vi "OutputArm.vi"() -> ()   [LabVIEW 2020]
uses:
  GlobalArm.vi
  TAI_Motor.vi
  GlobalDriverStationData.vi
panel:
  in  "Wrist Torque Compensation":dbl=1.0
  in  "Elbow Torque Compensation":dbl=1.0
  in  "Shoulder Torque Compensation":dbl=1.0
  in  "Shoulder Overrided State":enum16{"Safety", "Travelling", "Positioning"}(ring)
  in  "Elbow Overrided State":enum16{"Safety", "Travelling", "Positioning"}(ring)
  in  "Wrist Overrided State":enum16{"Safety", "Travelling", "Positioning"}(ring)
  in  "Wrist S-Curve Strength":dbl=4.0
  in  "Wrist Acceleration (deg/s^2)":dbl=300.0
  in  "Wrist Cruise Velocity (deg/s)":dbl=60.0
  in  "Wrist Override (deg)":dbl
  in  "Override Wrist State Machine":bool
  out "Wrist Position (deg)":dbl
  out "Wrist Position":cluster{dbl, "Interlock Output":dbl}(graph)
  out "Wrist Velocity":cluster{dbl}(graph)
  in  "Wrist Positioning PID Parameters":T1={"Kp"=0.0, "Ki"=0.0, "Kd"=0.0, "Kf (don't use)"=0.0, "I-Zone"=10.0} {"Kd" min=0.0; "Ki" min=0.0; "Kp" min=0.0}
  in  "Wrist Travelling PID Parameters":T1={"Kp"=0.0, "Ki"=0.0, "Kd"=0.0, "Kf (don't use)"=0.0, "I-Zone"=10.0} {"Kd" min=0.0; "Ki" min=0.0; "Kp" min=0.0}
  in  "Shoulder S-Curve Strength":dbl=4.0
  in  "Shoulder Acceleration (deg/s^2)":dbl=300.0
  in  "Shoulder Cruise Velocity (deg/s)":dbl=60.0
  in  "Shoulder Override (deg)":dbl
  in  "Override Shoulder State Machine":bool
  out "Shoulder Position (deg)":dbl
  out "Shoulder Position":cluster{dbl, "Interlock Output":dbl}(graph)
  out "Shoulder Velocity":cluster{dbl}(graph)
  in  "Shoulder Positioning PID Parameters":T1={"Kp"=0.0, "Ki"=0.0, "Kd"=0.0, "Kf (don't use)"=0.0, "I-Zone"=10.0} {"Kd" min=0.0; "Ki" min=0.0; "Kp" min=0.0}
  in  "Shoulder Travelling PID Parameters":T1={"Kp"=0.0, "Ki"=0.0, "Kd"=0.0, "Kf (don't use)"=0.0, "I-Zone"=10.0} {"Kd" min=0.0; "Ki" min=0.0; "Kp" min=0.0}
  in  "Elbow Override (deg)":dbl
  in  "Override Elbow State Machine":bool
  out "Elbow Position":cluster{dbl, "Interlock Output":dbl}(graph)
  out "Elbow Position (deg)":dbl
  out "Elbow Velocity":cluster{dbl}(graph)
  in  "Plot Joint Positions":bool
  in  "Elbow Positioning PID Parameters":T1={"Kp"=inf, "Ki"=0.0, "Kd"=0.0, "Kf (don't use)"=0.0, "I-Zone"=10.0} {"Kd" min=0.0; "Ki" min=0.0; "Kp" min=0.0}
  in  "Elbow Travelling PID Parameters":T1={"Kp"=0.0, "Ki"=0.0, "Kd"=0.0, "Kf (don't use)"=0.0, "I-Zone"=10.0} {"Kd" min=0.0; "Ki" min=0.0; "Kp" min=0.0}
  in  "Elbow S-Curve Strength":dbl=4.0
  in  "Elbow Acceleration (deg/s^2)":dbl=300.0
  in  "Elbow Cruise Velocity (deg/s)":dbl=60.0
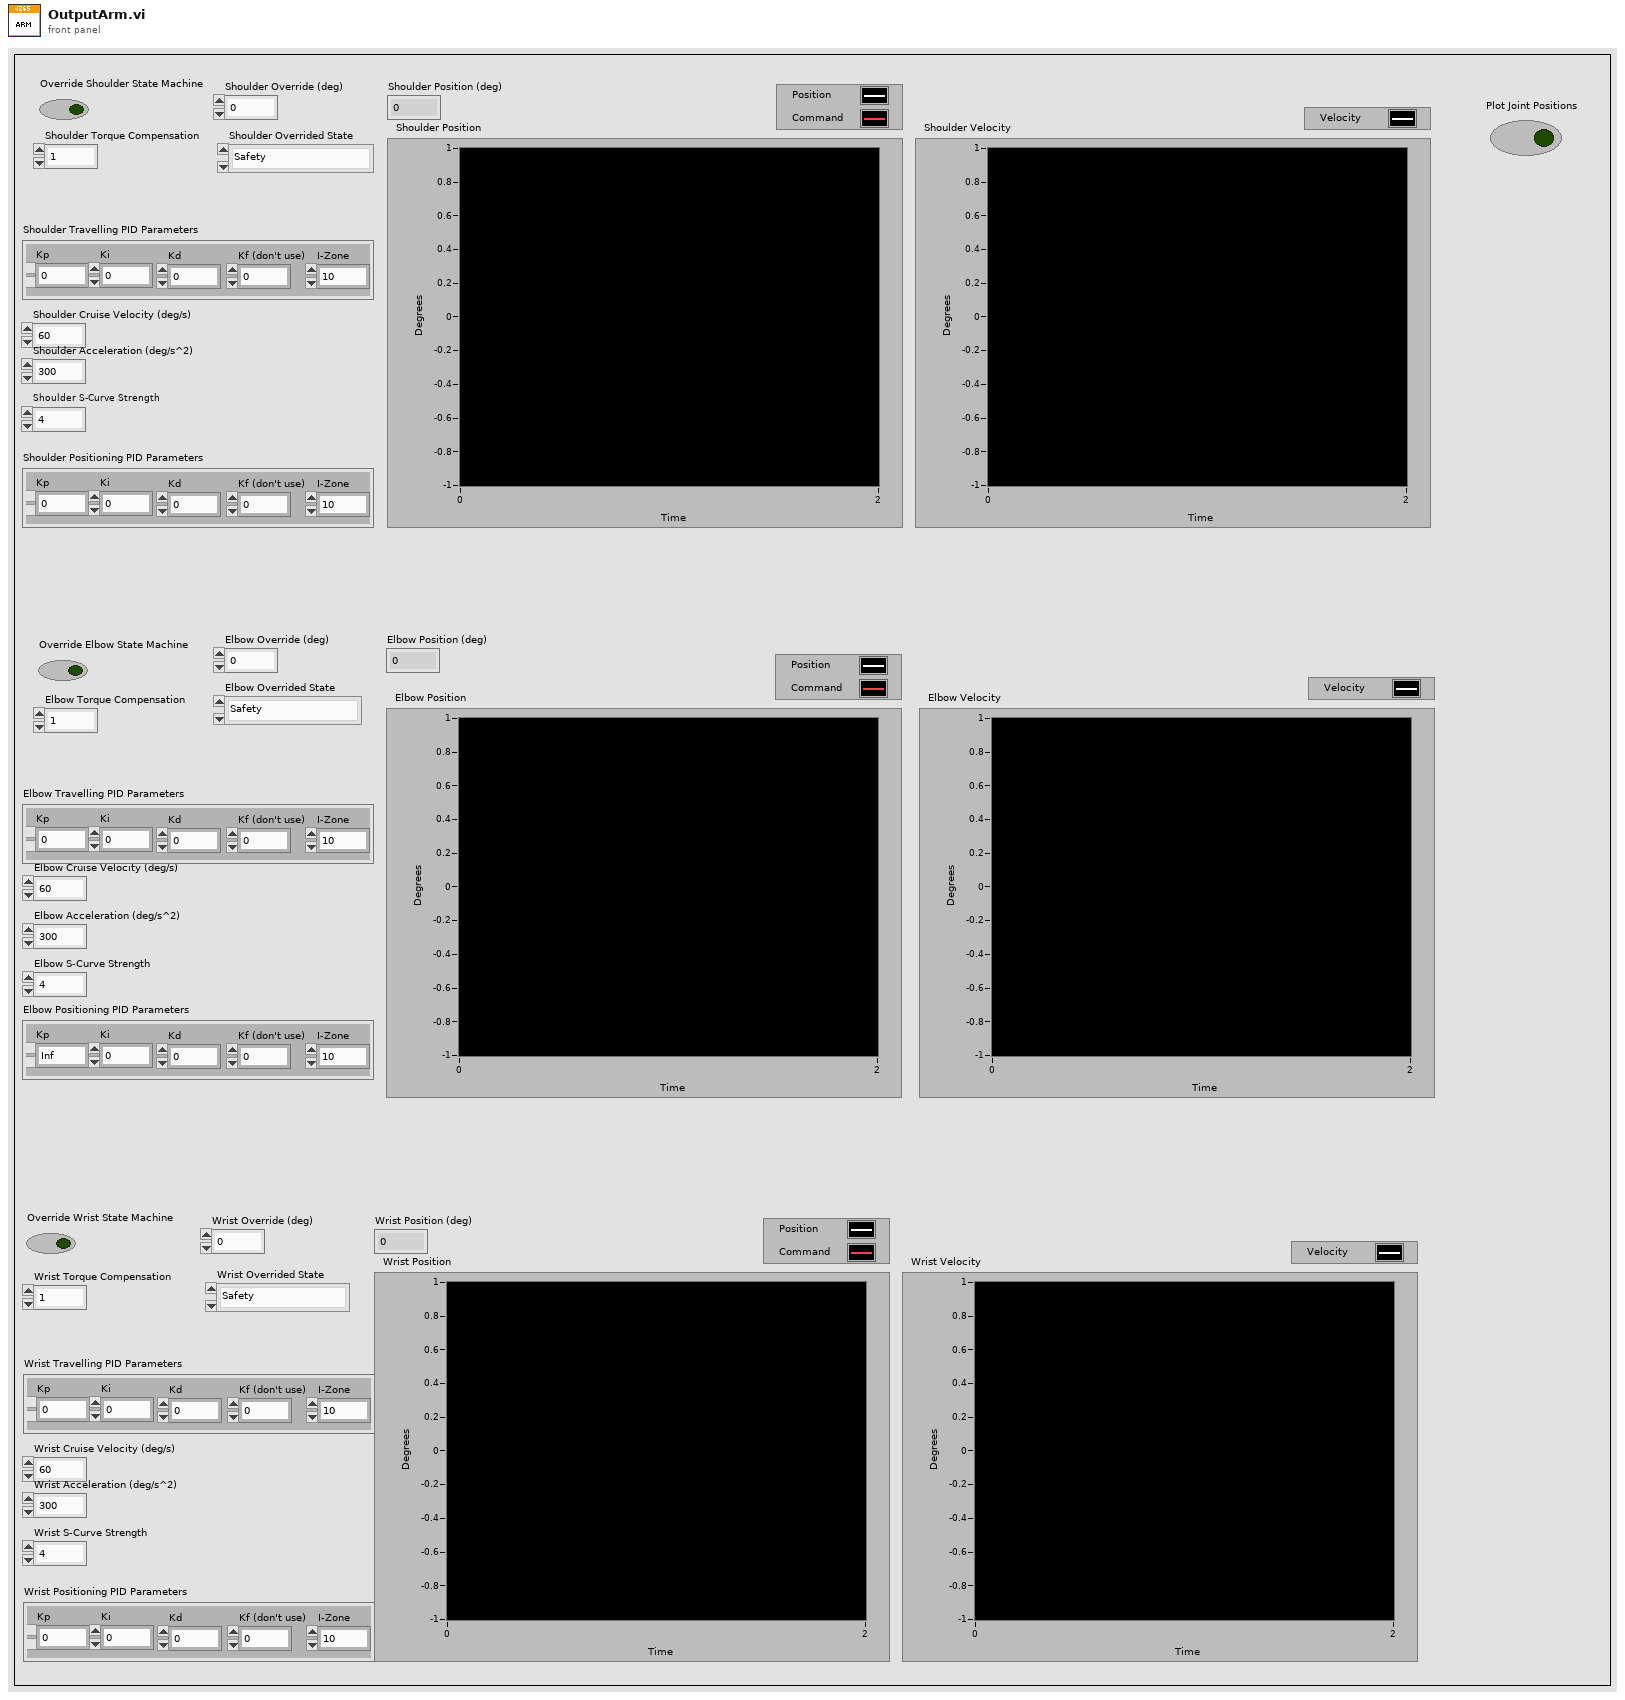
[diagram p1: front panel]
types:
  T1 = cluster{"Kp":dbl, "Ki":dbl, "Kd":dbl, "Kf (don't use)":dbl, "I-Zone":dbl}
  T2 = typedef "WPI_MotorControlDeviceRef.ctl" = cluster{"DeviceStatus":errorcluster, "Type":T3, "PWM":cluster{"PWM Channel":T4, "DeadBand":T5}, "CAN":cluster{"Device Number":u8, "SetOutput VI Ref":variant, "GetOutput VI Ref":variant, "Enable VI Ref":variant, "Disable VI Ref":variant, "Data":variant}, "Invert":bool, "DIO PWM":cluster{"PWM \"Enable\" Channel":T4, "DIOChannel":T6, "PWM Rate":dbl}}
  T3 = typedef "WPI_MotorControlType.ctl" = enum16{"PWM", "CAN", "DIO PWM"}
  T4 = typedef "FPGA_DIOPWMChannel.ctl" = enum8{"PWM 0", "PWM 1", "PWM 2", "PWM 3", "PWM 4", "PWM 5", "PWM 6", "PWM 7", "PWM 8", "PWM 9", "PWM MXP 0", "PWM MXP 1", "PWM MXP 2", "PWM MXP 3", "PWM MXP 4", "PWM MXP 5", "PWM MXP 6", "PWM MXP 7", "PWM MXP 8", "PWM MXP 9", "Invalid"}
  T5 = typedef "WPI_PWMDeadband.ctl" = cluster{"Name":string, "maxPositivePwm":i32, "minPositivePwm":i32, "centerPwm":i32, "maxNegativePwm":i32, "minNegativePwm":i32, "angularRange":u16}
  T6 = typedef "FPGA_DIOChannel.ctl" = enum8{"DIO 0", "DIO 1", "DIO 2", "DIO 3", "DIO 4", "DIO 5", "DIO 6", "DIO 7", "DIO 8", "DIO 9", "DIO MXP 0", "DIO MXP 1", "DIO MXP 2", "DIO MXP 3", "DIO MXP 4", "DIO MXP 5", "DIO MXP 6", "DIO MXP 7", "DIO MXP 8", "DIO MXP 9", "DIO MXP 10", "DIO MXP 11", "DIO MXP 12", "DIO MXP 13", "DIO MXP 14", "DIO MXP 15", "SPI Port CS1", "SPI Port CS2", "SPI Port CS3", "SPI Port MISO", "SPI Port MOSI", "Invalid"}
  T7 = enum16{"No Changed Output", "New Normal Output", "New Testing Output"}
  T8 = cluster{"Position (deg)":dbl, "OUT_Shoulder_Goal (deg)":dbl}
  T9 = cluster{"Position (deg)":dbl, "OUT_Wrist_Goal (deg)":dbl}
  T10 = cluster{"Position (deg)":dbl, "OUT_Elbow_Goal (deg)":dbl}
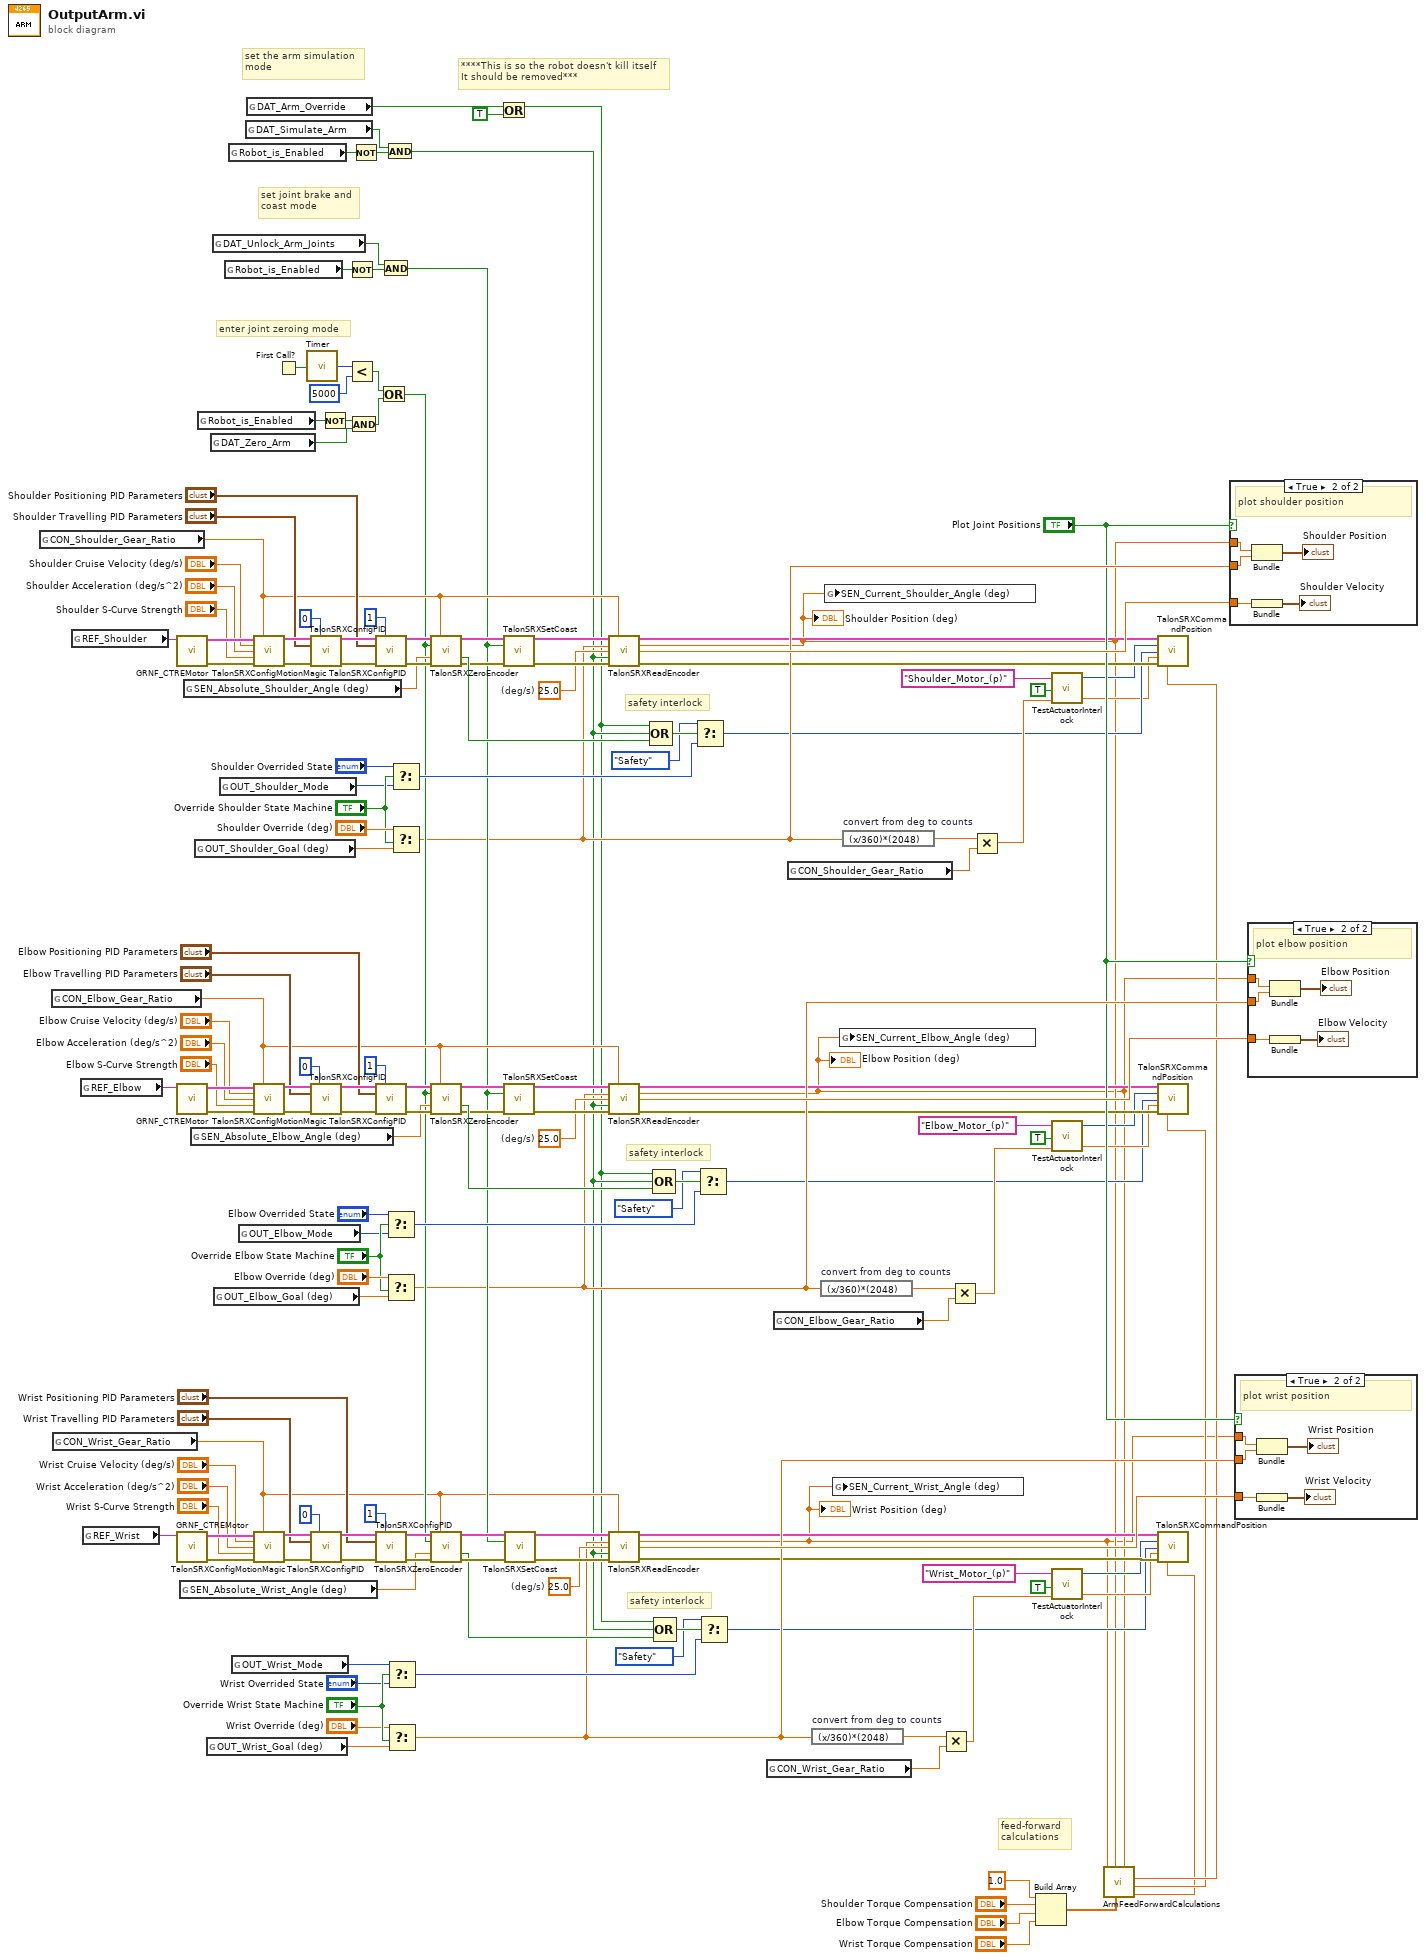
[diagram p0: block diagram]
diagram:
  w39 = 25.0  # (deg/s)
  w91 = 25.0  # (deg/s)
  w113 = 25.0  # (deg/s)
  # "****This is so the robot doesn't kill itself\nIt should be removed***"
  # "feed-forward\ncalculations"
  # "set the arm simulation\nmode"
  # "safety interlock"
  # "safety interlock"
  # "safety interlock"
  # "enter joint zeroing mode"
  # "set joint brake and\ncoast mode"
  n1 = global read "GlobalArm.vi" "CON_Shoulder_Gear_Ratio"() -> (w115:dbl)
  n2 = global read "GlobalArm.vi" "CON_Elbow_Gear_Ratio"() -> (w82:dbl)
  n3 = global read "GlobalArm.vi" "CON_Wrist_Gear_Ratio"() -> (w50:dbl)
  n4 = global read "GlobalArm.vi" "REF_Shoulder"() -> (w162:string)
  n5 = global read "GlobalArm.vi" "REF_Elbow"() -> (w88:string)
  n6 = global read "GlobalArm.vi" "REF_Wrist"() -> (w69:string)
  n7 = call "GRNF_CTREMotor.vi"("RefNum Name"=w162) -> ("Error"=w161:errorcluster, "Device Reference"=w134:T2)  [unwired: 5 in]
  n8 = call "GRNF_CTREMotor.vi"("RefNum Name"=w88) -> ("Error"=w111:errorcluster, "Device Reference"=w104:T2)  [unwired: 5 in]
  n9 = call "GRNF_CTREMotor.vi"("RefNum Name"=w69) -> ("Error"=w67:errorcluster, "Device Reference"=w77:T2)  [unwired: 5 in]
  n10 = global read "GlobalArm.vi" "SEN_Absolute_Wrist_Angle (deg)"() -> (w51:dbl)
  n11 = global read "GlobalArm.vi" "SEN_Absolute_Shoulder_Angle (deg)"() -> (w120:dbl)
  n12 = global read "GlobalArm.vi" "SEN_Absolute_Elbow_Angle (deg)"() -> (w97:dbl)
  n13 = global read "GlobalArm.vi" "OUT_Shoulder_Goal (deg)"() -> (w160:dbl)
  n14 = global read "GlobalDriverStationData.vi" "Robot_is_Enabled"() -> (w151:bool)
  n15 = global read "GlobalArm.vi" "OUT_Wrist_Goal (deg)"() -> (w49:dbl)
  n16 = global read "GlobalArm.vi" "DAT_Zero_Arm"() -> (w143:bool)
  n17 = global read "GlobalArm.vi" "DAT_Unlock_Arm_Joints"() -> (w140:bool)
  n18 = global read "GlobalArm.vi" "OUT_Elbow_Goal (deg)"() -> (w110:dbl)
  n19 = global read "GlobalArm.vi" "OUT_Shoulder_Mode"() -> (w46:enum16{"Safety", "Travelling", "Positioning"})
  n20 = global read "GlobalDriverStationData.vi" "Robot_is_Enabled"() -> (w142:bool)
  n21 = global read "GlobalDriverStationData.vi" "Robot_is_Enabled"() -> (w30:bool)
  n22 = global read "GlobalArm.vi" "OUT_Wrist_Mode"() -> (w41:enum16{"Safety", "Travelling", "Positioning"})
  n23 = global read "GlobalArm.vi" "OUT_Elbow_Mode"() -> (w44:enum16{"Safety", "Travelling", "Positioning"})
  n24 = global read "GlobalArm.vi" "DAT_Simulate_Arm"() -> (w28:bool)
  n25 = global read "GlobalArm.vi" "DAT_Arm_Override"() -> (w58:bool)
  n26 = call "TalonSRXConfigMotionMagic.vi"("Device Reference (in)"=w134, "Gear Ratio"=w115, "Cruise Velocity (deg/s)"="Shoulder Cruise Velocity (deg/s)", "Acceleration (deg/s^2)"="Shoulder Acceleration (deg/s^2)", "S-Curve Strength"="Shoulder S-Curve Strength", "Error (in)"=w161) -> ("Device Reference (out)"=w130:T2, "Error (out)"=w129:errorcluster)  [unwired: 8 in]
  n27 = call "TalonSRXConfigMotionMagic.vi"("Device Reference (in)"=w104, "Gear Ratio"=w82, "Cruise Velocity (deg/s)"="Elbow Cruise Velocity (deg/s)", "Acceleration (deg/s^2)"="Elbow Acceleration (deg/s^2)", "S-Curve Strength"="Elbow S-Curve Strength", "Error (in)"=w111) -> ("Device Reference (out)"=w103:T2, "Error (out)"=w102:errorcluster)  [unwired: 8 in]
  n28 = call "TalonSRXConfigMotionMagic.vi"("Device Reference (in)"=w77, "Gear Ratio"=w50, "Cruise Velocity (deg/s)"="Wrist Cruise Velocity (deg/s)", "Acceleration (deg/s^2)"="Wrist Acceleration (deg/s^2)", "S-Curve Strength"="Wrist S-Curve Strength", "Error (in)"=w67) -> ("Device Reference (out)"=w76:T2, "Error (out)"=w66:errorcluster)  [unwired: 8 in]
  n29 = First Call?() -> (First Call?: T/F=w156:bool)
  n30 = call "Timer.vi"("Reset Timer"=w156) -> ("Time (ms)"=w155:u32)
  n31 = call "TalonSRXConfigPID.vi"("Device Reference (in)"=w130, "PID Slot"=0 ("slotIdx"), "PID Parameters"="Shoulder Travelling PID Parameters", "Error (in)"=w129) -> ("Device Reference (out)"=w125:T2, "Error (out)"=w124:errorcluster)  [unwired: 10 in]
  n32 = call "TalonSRXConfigPID.vi"("Device Reference (in)"=w103, "PID Slot"=0 ("slotIdx"), "PID Parameters"="Elbow Travelling PID Parameters", "Error (in)"=w102) -> ("Device Reference (out)"=w101:T2, "Error (out)"=w100:errorcluster)  [unwired: 10 in]
  n33 = call "TalonSRXConfigPID.vi"("Device Reference (in)"=w76, "PID Slot"=0 ("slotIdx"), "PID Parameters"="Wrist Travelling PID Parameters", "Error (in)"=w66) -> ("Device Reference (out)"=w75:T2, "Error (out)"=w65:errorcluster)  [unwired: 10 in]
  n34 = Not(x=w151) -> (.not. x?=w152:bool)
  n35 = Not(x=w142) -> (.not. x?=w141:bool)
  n36 = Less?(x=w155, y=u32 5000) -> (x < y?=w153:bool)
  n37 = And(x=w152, y=w143) -> (x .and. y?=w150:bool)
  n38 = Not(x=w30) -> (.not. x?=w29:bool)
  n39 = call "TalonSRXConfigPID.vi"("Device Reference (in)"=w125, "PID Slot"=1 ("slotIdx"), "PID Parameters"="Shoulder Positioning PID Parameters", "Error (in)"=w124) -> ("Device Reference (out)"=w122:T2, "Error (out)"=w121:errorcluster)  [unwired: 10 in]
  n40 = call "TalonSRXConfigPID.vi"("Device Reference (in)"=w101, "PID Slot"=1 ("slotIdx"), "PID Parameters"="Elbow Positioning PID Parameters", "Error (in)"=w100) -> ("Device Reference (out)"=w99:T2, "Error (out)"=w98:errorcluster)  [unwired: 10 in]
  n41 = call "TalonSRXConfigPID.vi"("Device Reference (in)"=w75, "PID Slot"=1 ("slotIdx"), "PID Parameters"="Wrist Positioning PID Parameters", "Error (in)"=w65) -> ("Device Reference (out)"=w74:T2, "Error (out)"=w64:errorcluster)  [unwired: 10 in]
  n42 = Or(x=w153, y=w150) -> (x .or. y?=w68:bool)
  n43 = And(x=w140, y=w141) -> (x .and. y?=w59:bool)
  n44 = And(x=w28, y=w29) -> (x .and. y?=w27:bool)
  n45 = Select(t="Elbow Overrided State", s="Override Elbow State Machine", f=w44) -> (s? t:f=w105:enum16{"Safety", "Travelling", "Positioning"})
  n46 = Select(t="Elbow Override (deg)", s="Override Elbow State Machine", f=w110) -> (s? t:f=w34:dbl)
  n47 = Select(t=w41, s="Override Wrist State Machine", f="Wrist Overrided State") -> (s? t:f=w40:enum16{"Safety", "Travelling", "Positioning"})
  n48 = Select(t="Wrist Override (deg)", s="Override Wrist State Machine", f=w49) -> (s? t:f=w33:dbl)
  n49 = Select(t="Shoulder Overrided State", s="Override Shoulder State Machine", f=w46) -> (s? t:f=w145:enum16{"Safety", "Travelling", "Positioning"})
  n50 = Select(t="Shoulder Override (deg)", s="Override Shoulder State Machine", f=w160) -> (s? t:f=w32:dbl)
  n51 = call "TalonSRXZeroEncoder.vi"("Device Reference (in)"=w122, "Gear Ratio"=w115, "Zeroing Trigger"=w68, "Absolute Angle (deg)"=w120, "Error (in)"=w121) -> ("Device Reference (out)"=w118:T2, "Currently Zeroing"=w119:bool, "Error (out)"=w117:errorcluster)  [unwired: 8 in]
  n52 = call "TalonSRXZeroEncoder.vi"("Device Reference (in)"=w99, "Gear Ratio"=w82, "Zeroing Trigger"=w68, "Absolute Angle (deg)"=w97, "Error (in)"=w98) -> ("Device Reference (out)"=w95:T2, "Currently Zeroing"=w96:bool, "Error (out)"=w94:errorcluster)  [unwired: 8 in]
  n53 = call "TalonSRXZeroEncoder.vi"("Device Reference (in)"=w74, "Gear Ratio"=w50, "Zeroing Trigger"=w68, "Absolute Angle (deg)"=w51, "Error (in)"=w64) -> ("Device Reference (out)"=w73:T2, "Currently Zeroing"=w57:bool, "Error (out)"=w63:errorcluster)  [unwired: 8 in]
  n54 = Or(x=w58, y=TRUE) -> (x .or. y?=w2:bool)
  n55 = call "TalonSRXSetCoast.vi"("Device Reference (in)"=w118, "Set Coast Mode"=w59, "Error (in)"=w117) -> ("Device Reference (out)"=w114:T2, "Error (out)"=w116:errorcluster)  [unwired: 11 in]
  n56 = call "TalonSRXSetCoast.vi"("Device Reference (in)"=w95, "Set Coast Mode"=w59, "Error (in)"=w94) -> ("Device Reference (out)"=w92:T2, "Error (out)"=w93:errorcluster)  [unwired: 11 in]
  n57 = call "TalonSRXSetCoast.vi"("Device Reference (in)"=w73, "Set Coast Mode"=w59, "Error (in)"=w63) -> ("Device Reference (out)"=w72:T2, "Error (out)"=w62:errorcluster)  [unwired: 11 in]
  n58 = call "TalonSRXReadEncoder.vi"("Device Reference (in)"=w114, "Gear Ratio"=w115, "Simulated Position Goal (deg)"=w32, "Simulated Velocity (deg/s)"=w113, "Simulate"=w27, "Error (in)"=w116) -> ("Device Reference (out)"=w26:T2, "Position (deg)"=w5:dbl, "Velocity (deg/s)"=w112:dbl, "Error (out)"=w25:errorcluster)  [unwired: 6 in]
  "Shoulder Position (deg)" <- w5
  n59 = call "TalonSRXReadEncoder.vi"("Device Reference (in)"=w92, "Gear Ratio"=w82, "Simulated Position Goal (deg)"=w34, "Simulated Velocity (deg/s)"=w91, "Simulate"=w27, "Error (in)"=w93) -> ("Device Reference (out)"=w17:T2, "Position (deg)"=w4:dbl, "Velocity (deg/s)"=w78:dbl, "Error (out)"=w16:errorcluster)  [unwired: 6 in]
  "Elbow Position (deg)" <- w4
  n60 = call "TalonSRXReadEncoder.vi"("Device Reference (in)"=w72, "Gear Ratio"=w50, "Simulated Position Goal (deg)"=w33, "Simulated Velocity (deg/s)"=w39, "Simulate"=w27, "Error (in)"=w62) -> ("Device Reference (out)"=w11:T2, "Position (deg)"=w3:dbl, "Velocity (deg/s)"=w35:dbl, "Error (out)"=w10:errorcluster)  [unwired: 6 in]
  "Wrist Position (deg)" <- w3
  n61 = Compound Arithmetic op=OR(w2, w27, w119) -> (w149:bool)
  n62 = Compound Arithmetic op=OR(w2, w27, w96) -> (w108:bool)
  n63 = Compound Arithmetic op=OR(w2, w27, w57) -> (w61:bool)
  n64 = Select(t=enum16{"Safety", "Travelling", "Positioning"}."Safety", s=w149, f=w145) -> (s? t:f=w22:enum16{"Safety", "Travelling", "Positioning"})
  n65 = Select(t=enum16{"Safety", "Travelling", "Positioning"}."Safety", s=w108, f=w105) -> (s? t:f=w12:enum16{"Safety", "Travelling", "Positioning"})
  n66 = Select(t=enum16{"Safety", "Travelling", "Positioning"}."Safety", s=w61, f=w40) -> (s? t:f=w6:enum16{"Safety", "Travelling", "Positioning"})
  n67 = global read "GlobalArm.vi" "CON_Wrist_Gear_Ratio"() -> (w37:dbl)
  n68 = global read "GlobalArm.vi" "CON_Elbow_Gear_Ratio"() -> (w107:dbl)
  n69 = global read "GlobalArm.vi" "CON_Shoulder_Gear_Ratio"() -> (w148:dbl)
  n70 = expression code="(x/360)*(2048)" "convert from deg to counts"(w33) -> (w38:dbl)
  n71 = expression code="(x/360)*(2048)" "convert from deg to counts"(w34) -> (w109:dbl)
  n72 = global write "GlobalArm.vi" "SEN_Current_Shoulder_Angle (deg)"(w5) -> ()
  n73 = global write "GlobalArm.vi" "SEN_Current_Wrist_Angle (deg)"(w3) -> ()
  n74 = global write "GlobalArm.vi" "SEN_Current_Elbow_Angle (deg)"(w4) -> ()
  n75 = expression code="(x/360)*(2048)" "convert from deg to counts"(w32) -> (w158:dbl)
  n76 = Multiply(x=w38, y=w37) -> (x*y=w36:dbl)
  n77 = Multiply(x=w109, y=w107) -> (x*y=w79:dbl)
  n78 = Multiply(x=w158, y=w148) -> (x*y=w157:dbl)
  n79 = Build Array(1.0 ("element"), "Shoulder Torque Compensation", "Elbow Torque Compensation", "Wrist Torque Compensation") -> (w139:dbl[])
  n80 = call-poly "TestActuatorInterlock.vi"("Normal Output"=w157, "Aux Trigger"=TRUE, "Actuator Name"="Shoulder_Motor_(p)") -> ("Interlocked Output"=w21:dbl, "Testing Mode"=w23:T7)  [unwired: 2 in]
  n81 = call-poly "TestActuatorInterlock.vi"("Normal Output"=w79, "Aux Trigger"=TRUE, "Actuator Name"="Elbow_Motor_(p)") -> ("Interlocked Output"=w13:dbl, "Testing Mode"=w14:T7)  [unwired: 2 in]
  n82 = call-poly "TestActuatorInterlock.vi"("Normal Output"=w36, "Aux Trigger"=TRUE, "Actuator Name"="Wrist_Motor_(p)") -> ("Interlocked Output"=w7:dbl, "Testing Mode"=w8:T7)  [unwired: 2 in]
  n83 = call "ArmFeedForwardCalculations.vi"("Motor Torque Compensation"=w139, "Wrist Pos (deg)"=w3, "Elbow Pos (deg)"=w4, "Shoulder Pos (deg)"=w5) -> ("Wrist Power [-1, 1]"=w9:dbl, "Elbow Power [-1. 1]"=w15:dbl, "Shoulder Power [-1, 1]"=w24:dbl)  [unwired: 5 in]
  n84 = call "TalonSRXCommandPosition.vi"("Device Reference (in)"=w26, "Testing Mode"=w23, "Control Mode"=w22, "Position (counts) or Testing Power"=w21, "Error (in)"=w25, "Feed Forward Power [-1, 1]"=w24) -> ()  [unwired: 10 in]
  n85 = call "TalonSRXCommandPosition.vi"("Device Reference (in)"=w17, "Testing Mode"=w14, "Control Mode"=w12, "Position (counts) or Testing Power"=w13, "Error (in)"=w16, "Feed Forward Power [-1, 1]"=w15) -> ()  [unwired: 10 in]
  n86 = call "TalonSRXCommandPosition.vi"("Device Reference (in)"=w11, "Testing Mode"=w8, "Control Mode"=w6, "Position (counts) or Testing Power"=w7, "Error (in)"=w10, "Feed Forward Power [-1, 1]"=w9) -> ()  [unwired: 10 in]
  n87 = case shown="True" "Plot Joint Positions" {
    tunnel: w5 -> [_ w167]
    tunnel: w32 -> [_ w166]
    tunnel: w112 -> [_ w165]
    frame False {
    }
    frame True {
      # "plot shoulder position"
      n88 = Bundle("Position (deg)"=w167, "OUT_Shoulder_Goal (deg)"=w166) -> (→"Shoulder Position":T8)  [unwired: 1 in]
      n89 = Bundle("Velocity (deg/s)"=w165) -> (→"Shoulder Velocity":cluster{"Velocity (deg/s)":dbl})  [unwired: 1 in]
    }
  }
  n90 = case shown="True" "Plot Joint Positions" {
    tunnel: w3 -> [_ w172]
    tunnel: w33 -> [_ w171]
    tunnel: w35 -> [_ w170]
    frame False {
    }
    frame True {
      # "plot wrist position"
      n91 = Bundle("Position (deg)"=w172, "OUT_Wrist_Goal (deg)"=w171) -> (→"Wrist Position":T9)  [unwired: 1 in]
      n92 = Bundle("Velocity (deg/s)"=w170) -> (→"Wrist Velocity":cluster{"Velocity (deg/s)":dbl})  [unwired: 1 in]
    }
  }
  n93 = case shown="True" "Plot Joint Positions" {
    tunnel: w4 -> [_ w177]
    tunnel: w34 -> [_ w176]
    tunnel: w78 -> [_ w175]
    frame False {
    }
    frame True {
      # "plot elbow position"
      n94 = Bundle("Position (deg)"=w177, "OUT_Elbow_Goal (deg)"=w176) -> (→"Elbow Position":T10)  [unwired: 1 in]
      n95 = Bundle("Velocity (deg/s)"=w175) -> (→"Elbow Velocity":cluster{"Velocity (deg/s)":dbl})  [unwired: 1 in]
    }
  }
